vi "Inputs Automo Global.vi"() -> ()   [LabVIEW 2014]
panel:
  in  "En nivel 1":bool
  in  "Levantamos el bote":bool
  in  "Rinse and repeat?":bool
  in  "Nos alejamos de la caja":bool
  in  "Dejamos caja":bool
  in  "Rotamos los x grados":bool
  in  "A distancia para recoger la caja":bool
  in  "Done picking up":bool
  in  "Estamos en el autozone":bool
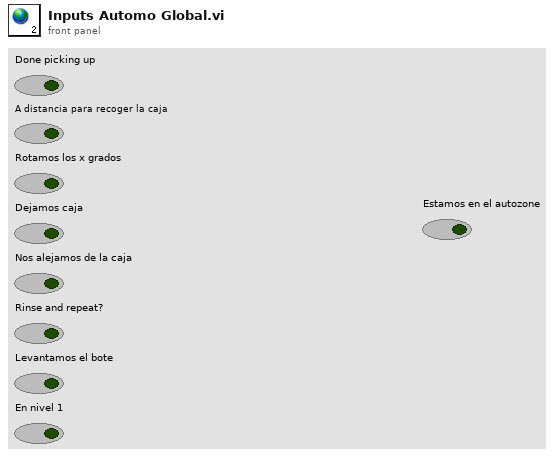
[diagram p1: front panel]
diagram:
